vi "Basic acquisition.vi"() -> ()   [LabVIEW 2009]
panel:
  in  "Acquisition type":i32(ring)=1 items=["JYMCD_ACQ_FORMAT_IMAGE", "JYMCD_ACQ_FORMAT_SCAN"]
  in  "Gain":i32
  in  "Integration time(ms)":i16=10
  in  "Select ADC":i32(ring) items=["JY_ADC_16_BIT", "JY_ADC_14_BIT", "JY_ADC_18_BIT"]
  out "Datas":i32[][](graph)
  in  "Shutter":bool
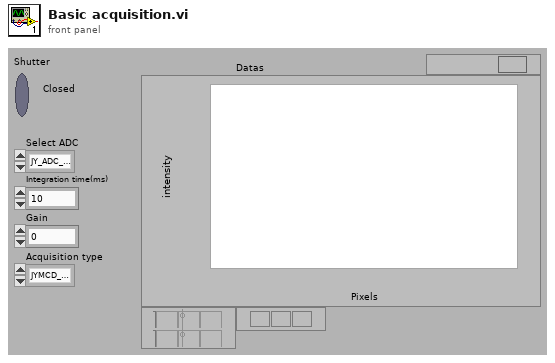
[diagram p1: front panel]
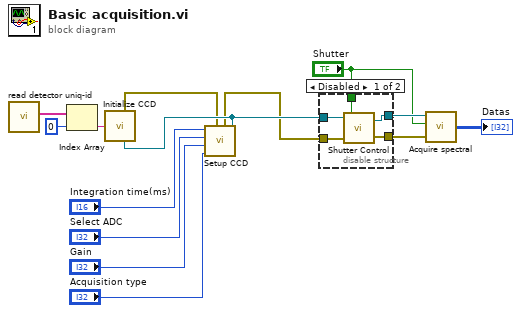
[diagram p0: block diagram]
diagram:
  n1 = call "read detector uniq-id.vi"() -> ("UniqueID"=w14:string[])  [unwired: 6 out]
  n2 = Index Array(array=w14, index=0) -> (element=w12:string)
  n3 = call "Initialize CCD.vi"("Unique id:"=w12) -> ("JYCCDLib.IJYCCDReqd"=w7:refnum<k7>, "sortie d'erreur"=w6:errorcluster)  [unwired: 6 out]
  n4 = call "Setup CCD.vi"("JYCCDLib.IJYCCDReqd"=w7, "entrée d'erreur (pas d'erreur)"=w6, "Acquisition type"="Acquisition type", "Gain"="Gain", "Select ADC"="Select ADC", "Integration time(ms)"="Integration time(ms)") -> ("sortie d'erreur"=w5:errorcluster)  [unwired: 2 in, 1 out]
  n5 = disable-structure shown="Disabled" {
    disable-tunnel: [w19 w21] -> w11
    disable-tunnel: "Shutter" -> [w18 _]
    disable-tunnel: [w17 w20] -> w9
    disable-tunnel: w7 -> [w16 w21]
    disable-tunnel: w5 -> [w15 w20]
    frame #0 {
      n6 = call "Shutter Control.vi"("input error"=w15, "Shutter"=w18, "JYCCDLib.IJYCCDReqd"=w16) -> ("error out"=w17:errorcluster, "JYCCDLib.IJYCCDReqd 2"=w19:refnum<k7>)
    }
    frame #1 {
    }
  }
  n7 = call "Acquire spectral.vi"("error in"=w9, "ShutterOpen"="Shutter", "JYCCDLib.IJYCCDReqd"=w11) -> ("Datas"=→"Datas":i32[][])  [unwired: 3 out]
